vi "Configure RangeMin.vi"(8 "error in (no error)":errorcluster, 9 "RangeMin":dbl, 10 "AxisNumber":u8, 11 "CS++Motor in":refnum<class "CS++Motor.lvclass">) -> (0 "error out":errorcluster, 3 "CS++Motor out":refnum<class "CS++Motor.lvclass">)   [LabVIEW 2015, in "CS++Motor.lvlib" / "CS++Motor.lvclass"]
doc: "Configures the minimum position that is allowed for a move of the axis."
uses:
  CS++Motor.lvclass
  CS++Motor.lvclass/CS++Motor.ctl
  CSPP_Core/Classes/CS++ProcessVariables/ProcessVariable/PV.lvclass
  PV-Enum-n.ctl
  CSPP_Core/Classes/CS++ProcessVariables/ProcessVariable/PV.lvclass/PV.ctl
  CSPP_Core/Classes/CS++ProcessVariables/ProcessVariable/Write Data.vi
  CSPP_Core/Classes/CS++ProcessVariables/ProcessVariable/Write Timestamp.vi
  CSPP_Core/Classes/CS++ProcessVariables/ProcessVariable/Write Quality.vi
  CSPP_Core/Classes/CS++ProcessVariables/ProcessVariable/Write status.vi
  CSPP_Core/Classes/CS++ProcessVariables/PVConnection/PVConnection.lvclass
  CSPP_Core/Libraries/Utilities/CS++Utilities.lvlib
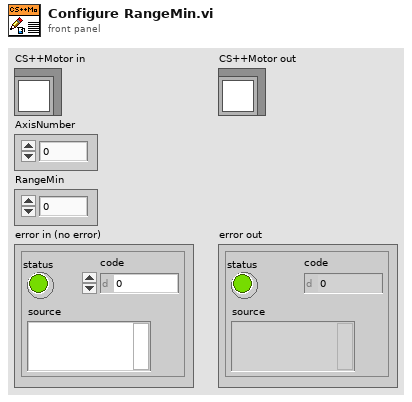
[diagram p1: front panel]
types:
  T1 = typedef "CS++Motor.lvlib/CS++Motor.lvclass/PV-Enum-n.ctl" = enum16{"LogicalName", "PhysicalName", "Active?", "unit", "SetPosition", "ActPosition", "StartVelocity", "StopVelocity", "Acceleration", "RangeMin", "RangeMax", "Scaling", "Status"}
  T2 = cluster{"LogicalName":string, "PhysicalName":string, "Active?":bool, "unit":string, "Scaling":dbl, "SetPosition":dbl, "ActPosition":dbl, "StartVelocity":dbl, "StopVelocity":dbl, "Acceleration":dbl, "RangeMin":dbl, "RangeMax":dbl, "Status":u32}[]
  T3 = cluster{"LogicalName":string, "PhysicalName":string, "Active?":bool, "unit":string, "Scaling":dbl, "SetPosition":dbl, "ActPosition":dbl, "StartVelocity":dbl, "StopVelocity":dbl, "Acceleration":dbl, "RangeMin":dbl, "RangeMax":dbl, "Status":u32}
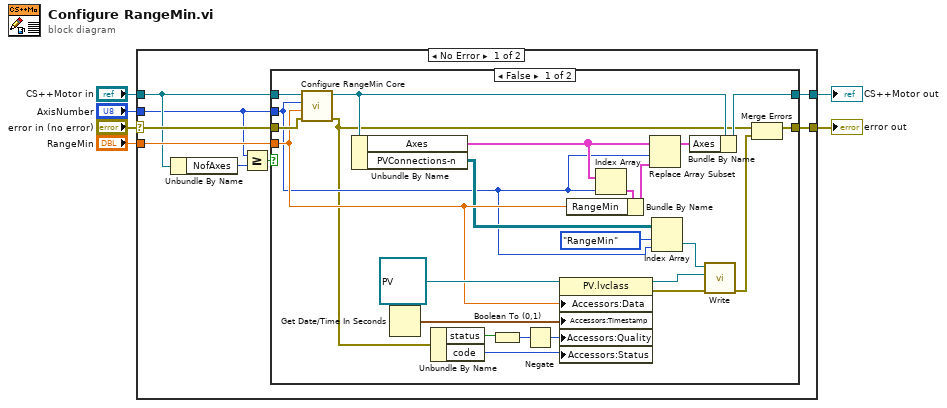
[diagram p0: block diagram]
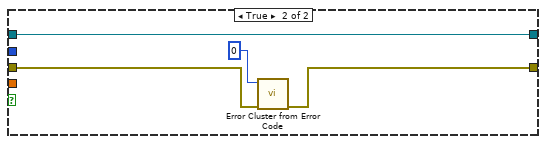
[diagram p2: hidden frame]
diagram:
  n1 = case shown="No Error" "error in (no error)" {
    selector: "error in (no error)" -> [w14 w44]
    tunnel: [w10 w44] -> w5
    tunnel: [w12 w43] -> w6
    tunnel: "CS++Motor in" -> [w11 w43]
    tunnel: "AxisNumber" -> [w9 _]
    tunnel: "RangeMin" -> [w13 _]
    frame No Error {
      n2 = Unbundle By Name(w11) -> ("NofAxes"=w8:u8)
      n3 = Greater Or Equal?(x=w9, y=w8) -> (x >= y?=w7:bool)
      n4 = case shown="False" w7 {
        tunnel: w14 -> [w38 w41]
        tunnel: w9 -> [w19 _]
        tunnel: w13 -> [w24 _]
        tunnel: [w32 w42] -> w12
        tunnel: w11 -> [w36 w42]
        tunnel: [w17 w40] -> w10
        frame False {
          n5 = call-dynamic "Configure RangeMin Core.vi"("error in (no error)"=w38, "RangeMin"=w24, "AxisNumber"=w19, "CS++Motor in"=w36) -> ("error out"=w16:errorcluster, "CS++Motor out"=w37:refnum<class "CS++Motor.lvclass">)  [unwired: 6 in]
          n6 = Unbundle By Name(w37) -> ("Axes"=w35:T2, "PVConnections-n"=w21:refnum<class "PVConnection.lvclass">[][])
          n7 = Get Date/Time In Seconds() -> (seconds since 1Jan1904=w30:timestamp)
          n8 = Unbundle By Name(w16) -> ("status"=w28:bool, "code"=w26:i32)
          n9 = Boolean To (0,1)(Boolean=w28) -> (0, 1=w27:i16)
          n10 = Negate(x=w27) -> (-x=w25:i16)
          n11 = property class="PV.lvclass"(reference=refnum<class "PV.lvclass"> refnum ("PV"), "Accessors:Data"=w24, "Accessors:Timestamp"=w30, "Accessors:Quality"=w25, "Accessors:Status"=w26) -> (reference out=w23:refnum<class "PV.lvclass">, error out=w22:errorcluster)  [unwired: 1 in]
          n12 = Index Array(array=w35, index=w19) -> (element=w34:T3)
          n13 = Bundle By Name(cluster=w34, "RangeMin"=w24) -> (w33:T3)
          n14 = Replace Array Subset(array=w35, new element=w33, index=w19) -> (w31:T2)
          n15 = Index Array(array=w21, index (row)=PV-Enum-n."RangeMin" ("PV-Enum-n"), index (col)=w19) -> (element=w20:refnum<class "PVConnection.lvclass">)
          n16 = Bundle By Name(cluster=w37, "Axes"=w31) -> (w32:refnum<class "CS++Motor.lvclass">)
          n17 = call "Write.vi"("error in (no error)"=w22, "PV"=w23, "PVConnection in"=w20) -> ("error out"=w18:errorcluster)  [unwired: 7 in, 1 out]
          n18 = Merge Errors(w16, w18) -> (w17:errorcluster)
        }
        frame True {
          n19 = call "Error Cluster from Error Code.vi"("Error In"=w41, "Error Code (0)"=0) -> ("Error Out"=w40:errorcluster)  [unwired: 9 in]
        }
      }
    }
    frame Error {
    }
  }
  "error out" <- w5
  "CS++Motor out" <- w6
